vi "Check Save Frame.vi"(6 "Main UI":refnum<vi>, 8 "error in (no error)":errorcluster, 11 "SB App in":refnum<class "SB App.lvclass">) -> (0 "error out":errorcluster, 3 "SB App out":refnum<class "SB App.lvclass">)   [LabVIEW 2020, in "SB App.lvlib" / "SB App.lvclass"]
uses:
  SB App.lvclass
  SB App.lvclass/SB App.ctl
  SquareBattle/Game/Game.lvclass
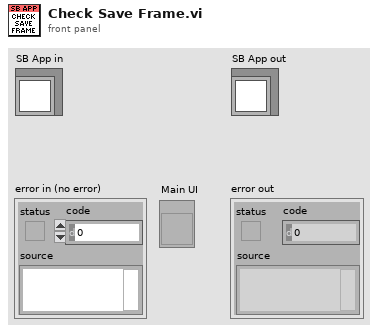
[diagram p1: front panel]
types:
  T1 = typedef "imagedata.ctl" = cluster{"image type":i32, "image depth":i32, "image":u8[], "mask":u8[], "colors":u32[], "Rectangle":cluster{"left":i16, "top":i16, "right":i16, "bottom":i16}}
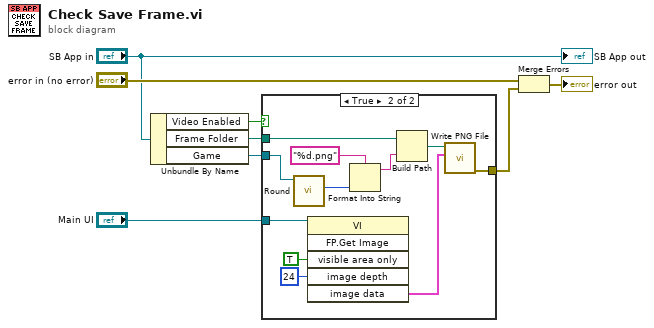
[diagram p0: block diagram]
diagram:
  n1 = Unbundle By Name("SB App in") -> ("Video Enabled"=w3:bool, "Frame Folder"=w4:path, "Game"=w5:refnum<class "Game.lvclass">)
  n2 = case shown="True" w3 {
    tunnel: "Main UI" -> [_ w19]
    tunnel: w5 -> [_ w15]
    tunnel: w4 -> [_ w12]
    tunnel: [_ w9] -> w1
    frame False {
    }
    frame True {
      n3 = call "Round.vi"("Game in"=w15) -> ("Round"=w14:u32)  [unwired: 8 in, 2 out]
      n4 = invoke class="VI" method="FP.Get Image"(reference=w19, "visible area only"=TRUE ("Visible Area Only"), "image depth"=24 ("Image Depth")) -> ("image data"=w16:T1)  [unwired: 3 in, 5 out]
      n5 = Format Into String(format string="%d.png", w14) -> (resulting string=w11:string)  [unwired: 2 in, 1 out]
      n6 = Build Path(base path=w12, name or relative path=w11) -> (appended path=w10:path)
      n7 = call <vilib>:"Write PNG File.vi"("image data"=w16, "path to PNG file"=w10) -> ("error out"=w9:errorcluster)  [unwired: 8 in, 1 out]
    }
  }
  n8 = Merge Errors("error in (no error)", w1) -> (→"error out":errorcluster)
  "SB App out" <- "SB App in"
